vi "Get NumSegments.vi"(8 "error in (no error)":errorcluster, 11 "TreeNode in":refnum<class "TreeNode.lvclass">) -> (0 "error out":errorcluster, 2 "NumSegments":i32, 3 "TreeNode out":refnum<class "TreeNode.lvclass">)   [LabVIEW 2010, in "MDSplus.lvlib" / "TreeNode.lvclass"]
uses:
  <vilib>/MDSplus/Classes/Data_Class/TreeNode_Class/TreeNode.lvclass
  <vilib>/MDSplus/MDSobjectsLVShr.dll
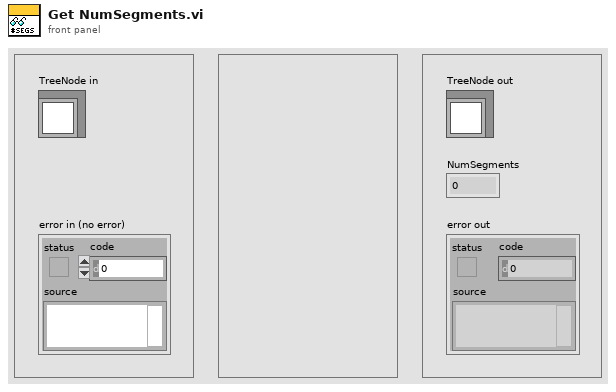
[diagram p1: front panel]
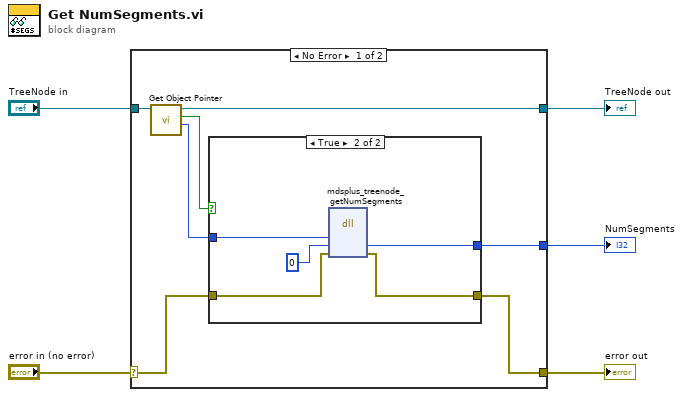
[diagram p0: block diagram]
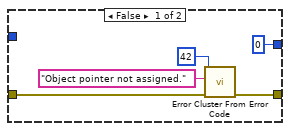
[diagram p2: hidden frame]
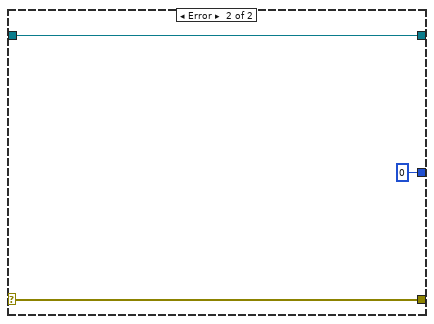
[diagram p3: hidden frame]
diagram:
  n1 = case shown="No Error" "error in (no error)" {
    selector: "error in (no error)" -> [w8 w25]
    tunnel: [w7 w25] -> w4
    tunnel: [w9 w24] -> w2
    tunnel: "TreeNode in" -> [w10 w24]
    tunnel: [w6 0 ("numSegmentsOut")] -> w1
    frame No Error {
      n2 = call-dynamic "Get Object Pointer.vi"("Data in"=w10) -> ("Object Pointer"=w11:i64, "Assigned object pointer?"=w12:bool, "Data out"=w9:refnum<class "TreeNode.lvclass">)  [unwired: 8 in]
      n3 = case shown="True" w12 {
        tunnel: w11 -> [_ w21]
        tunnel: w8 -> [w15 w20]
        tunnel: [w14 w19] -> w7
        tunnel: [0 ("numSegmentsOut") w18] -> w6
        frame False {
          n4 = call <vilib>:"Error Cluster From Error Code.vi"("error in (no error)"=w15, "error message (\"\")"="Object pointer not assigned." ("error message (\"\")"), "error code (0)"=42) -> ("error out"=w14:errorcluster)  [unwired: 6 in]
        }
        frame True {
          n5 = dll-call lib="C:/Program Files (x86)/National Instruments/LabVIEW 2012/vi.lib/MDSplus/MDSobjectsLVShr.dll" fn="mdsplus_treenode_getNumSegments"("lvTreeNodePtr"=w21, "numSegmentsOut"=0 ("floatOut"), "error"=w20) -> ("numSegmentsOut"=w18:i32, "error"=w19:errorcluster)  [unwired: 5 in, 2 out]
        }
      }
    }
    frame Error {
    }
  }
  "error out" <- w4
  "TreeNode out" <- w2
  "NumSegments" <- w1
